vi "Initialize.vi"(8 "error in":errorcluster, 10 "parameters":variant, 11 "Engine in":refnum<class "Engine Parent Editor Node.lvclass">) -> (0 "error out":errorcluster, 2 "summary":T2[](array[typedef]), 3 "data value reference":T1)   [LabVIEW 2013, in "PL Framework Configuration Tool.lvlib" / "Engine Parent Editor Node.lvclass"]
doc: "This Vi initializes the data of a node its default state.\nThe object is not created inside of this ViI, beacuase it is created from a File depending on user selection."
uses:
  Engine Parent Editor Node.lvclass
  <vilib>/NI/Configuration Framework/Node/Summary.ctl
  <vilib>/NI/Configuration Framework/Node/NodeRef.ctl
  <vilib>/NI/Configuration Framework/Node/NISE_CEF_Node.lvclass
  EngineTags/EngineTags.lvclass
  Engine Mappings/Engine Mappings.lvclass
  TBM Configuration Node/TBM Configuration Node.lvclass
  <vilib>/NI/Configuration Framework/NISE_CEF_TreeControl.lvlib
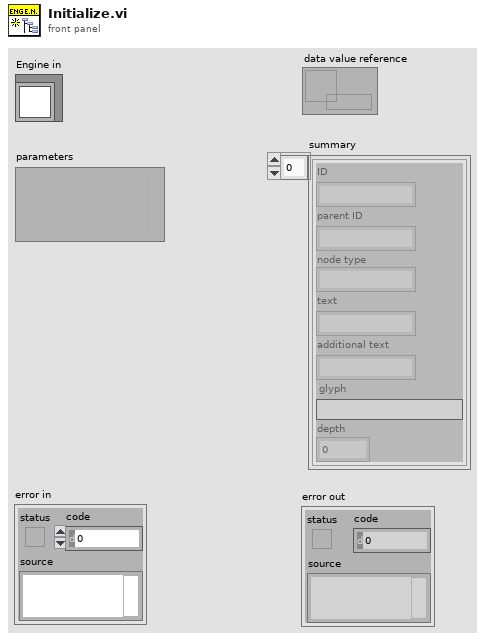
[diagram p1: front panel]
types:
  T1 = typedef "NISE_CEF_Node.lvclass/NodeRef.ctl" = refnum<data-value>
  T2 = typedef "NISE_CEF_Node.lvclass/Summary.ctl" = cluster{"ID":string, "parent ID":string, "node type":string, "text":string, "additional text":string, "glyph":string, "depth":i32}
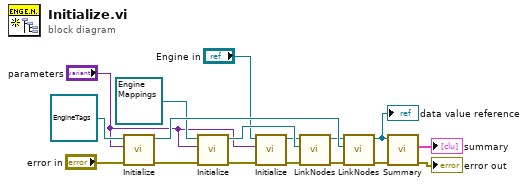
[diagram p0: block diagram]
diagram:
  n1 = call-dynamic "Initialize.vi"("error in"="error in", "parameters"="parameters", "node in"=refnum<class "EngineTags.lvclass"> refnum ("EngineTags.lvclass")) -> ("error out"=w8:errorcluster, "data value reference"=w12:T1)  [unwired: 6 in, 1 out]
  n2 = call-dynamic "Initialize.vi"("error in"=w8, "parameters"="parameters", "node in"=refnum<class "Engine Mappings.lvclass"> refnum ("PL Framework Configuration Tool.lvlib:Engine Mapping Viewer")) -> ("error out"=w5:errorcluster, "data value reference"=w7:T1)  [unwired: 6 in, 1 out]
  n3 = call-parent "Initialize.vi"("error in"=w5, "parameters"="parameters", "node in"="Engine in") -> ("error out"=w3:errorcluster, "data value reference"=w2:T1)  [unwired: 6 in, 1 out]
  n4 = call <vilib>:"LinkNodes.vi"("error in"=w3, "child in"=w7, "parent in"=w2) -> ("error out"=w10:errorcluster, "parent out"=w9:T1)  [unwired: 6 in, 1 out]
  n5 = call <vilib>:"LinkNodes.vi"("error in"=w10, "child in"=w12, "parent in"=w9) -> ("error out"=w17:errorcluster, "parent out"=w15:T1)  [unwired: 6 in, 1 out]
  "data value reference" <- w15
  n6 = call <vilib>:"Summary.vi"("error in"=w17, "node self ref"=w15) -> ("error out"=→"error out":errorcluster, "summary"=→"summary":T2[])  [unwired: 8 in]
